vi "CreatePrivateEvents.vi"(8 "error in (no error)":errorcluster, 11 "LockinDAQ":refnum<class "LockinDAQ.lvclass">) -> (0 "error out":errorcluster, 3 "LockinDAQ out":refnum<class "LockinDAQ.lvclass">)   [LabVIEW 2016, in "LockinDAQ.lvclass"]
doc: "---------------------------------------------------------------\nJKI State Machine Objects™\nhttp://jki.net/state-machine-objects/\nCopyright (C) 2005-2015, JKI <info@jki.net>\nALL RIGHTS RESERVEDJKI State Machine Objects (SMO) 1.0.0.4\nJKI - JKI\nCopyright (c) 2015, JKI"
uses:
  LockinDAQ.lvclass
  Typedefs/PrivateEvents--LockinDAQ.setAOconfig.ctl
  Typedefs/AO.config-array.ctl
  Typedefs/AO.config-cluster.ctl
  Typedefs/446xAO-enum.ctl
  Typedefs/PrivateEvents--LockinDAQ.setAIconfig.ctl
  Typedefs/AI.config-array.ctl
  Typedefs/AI.config-cluster.ctl
  Typedefs/AI.coupling-enum.ctl
  Typedefs/446xAI-enum.ctl
  Typedefs/PrivateEvents--LockinDAQ.setAO.ctl
  Typedefs/AO-cluster.ctl
  Typedefs/AO_Amp-array.ctl
  Typedefs/AO_DC-array.ctl
  Typedefs/AO_f-array.ctl
  Typedefs/AO_phi-array.ctl
  Typedefs/Function-array.ctl
  Typedefs/Function-enum.ctl
  Typedefs/PrivateEvents--LockinDAQ.setREF.ctl
  Typedefs/REF-cluster.ctl
  Typedefs/REF_f-array.ctl
  Typedefs/REF_phi-array.ctl
  Typedefs/PrivateEvents--LockinDAQ.setSampling.ctl
  Typedefs/Sampling.ctl
  Typedefs/PrivateEvents--LockinDAQ.setState.ctl
  Typedefs/Set State-enum.ctl
  LockinDAQ.lvclass/LockinDAQ.ctl
  <vilib>/JKI/JKI SMO/SMO/SMO.lvclass
panel:
  # "For instructions on how to use the JKI State Machine Objects, examples and video tutorials, visit:\nhttp://jki.net/state-machine-objects/\n\nJKI State Machine Objects™\nhttp://jki.net/state-machine-objects/\nCopyright (C) 2005-2015, JKI <info@jki.net>\nALL RIGHTS RESERVED"
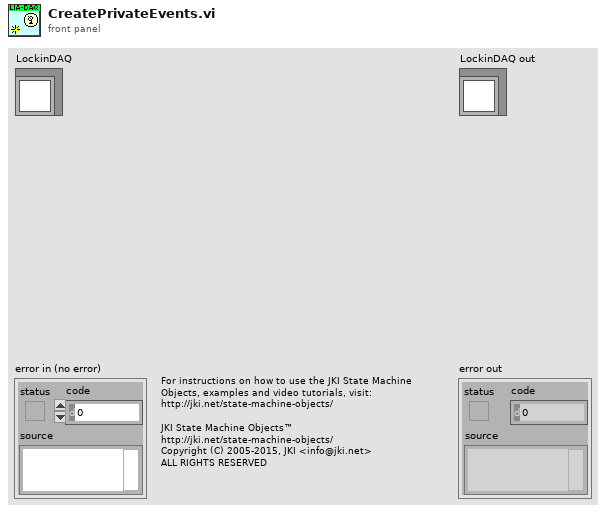
[diagram p1: front panel]
types:
  T1 = typedef "LockinDAQ.lvclass/PrivateEvents--LockinDAQ.setState.ctl" = cluster{"setState":T2}
  T2 = typedef "LockinDAQ.lvclass/Set State-enum.ctl" = enum16{"start", "stop", "reset"}
  T3 = typedef "LockinDAQ.lvclass/PrivateEvents--LockinDAQ.setSampling.ctl" = cluster{"sampling":T4, "sample mode":i32}
  T4 = typedef "Sampling.ctl" = cluster{"Fs":dbl, "#s":i32}
  T5 = typedef "LockinDAQ.lvclass/PrivateEvents--LockinDAQ.setREF.ctl" = cluster{"Channels: Lockin":T6}
  T6 = typedef "REF-cluster.ctl" = cluster{"REF f (Hz)":T7, "REF phi (°)":T8}
  T7 = typedef "REF_f-array.ctl" = dbl[]
  T8 = typedef "REF_phi-array.ctl" = dbl[]
  T9 = typedef "LockinDAQ.lvclass/PrivateEvents--LockinDAQ.setAO.ctl" = cluster{"Channels: AO":T10}
  T10 = typedef "AO-cluster.ctl" = cluster{"AO amp (V)":T11, "AO DC (V)":T12, "AO f (Hz)":T13, "AO phi (°)":T14, "function":T15, "I+":bool[]}
  T11 = typedef "AO_Amp-array.ctl" = dbl[]
  T12 = typedef "AO_DC-array.ctl" = dbl[]
  T13 = typedef "AO_f-array.ctl" = dbl[]
  T14 = typedef "AO_phi-array.ctl" = dbl[]
  T15 = typedef "Function-array.ctl" = T16[]
  T16 = typedef "Function-enum.ctl" = enum16{"Sine", "Triangle", "Square", "Sawtooth"}
  T17 = typedef "LockinDAQ.lvclass/PrivateEvents--LockinDAQ.setAIconfig.ctl" = cluster{"AI Configuration":T18}
  T18 = typedef "AI.config-array.ctl" = T19[]
  T19 = typedef "AI.config-cluster.ctl" = cluster{"AI.Coupling":T20, "AI.channels":tag, "AI.Range":T21}
  T20 = typedef "AI.coupling-enum.ctl" = enum16{"AC", "DC", "GND"}
  T21 = typedef "446xAI-enum.ctl" = enum16{"±0.316 V", "±1.00 V", "±3.16 V", "±10.0 V", "±31.6 V", "±42.4 V"}
  T22 = typedef "LockinDAQ.lvclass/PrivateEvents--LockinDAQ.setAOconfig.ctl" = cluster{"AO Configuration":T23}
  T23 = typedef "AO.config-array.ctl" = T24[]
  T24 = typedef "AO.config-cluster.ctl" = cluster{"AO.Range":T25, "AO.channels":tag}
  T25 = typedef "446xAO-enum.ctl" = enum16{"±0.1 V", "±1.0 V", "±10.0 V"}
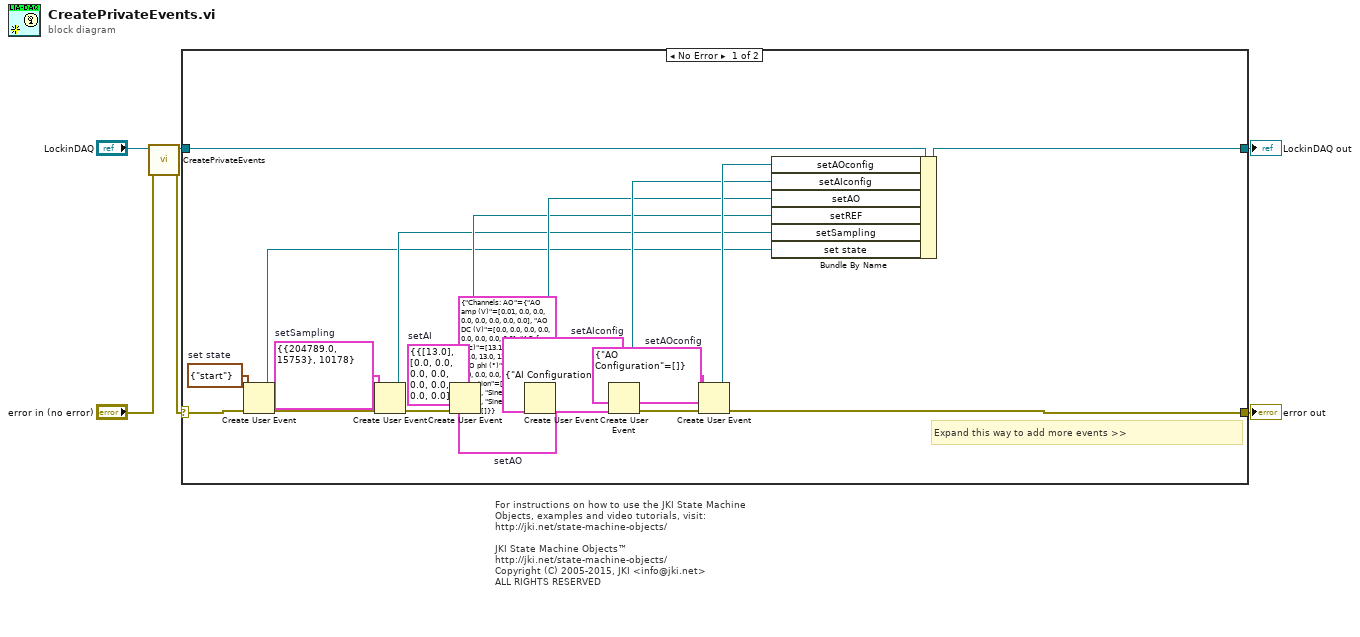
[diagram p0: block diagram]
diagram:
  # "For instructions on how to use the JKI State Machine Objects, examples and video tutorials, visit:\nhttp://jki.net/state-machine-objects/\n\nJKI State Machine Objects™\nhttp://jki.net/state-machine-objects/\nCopyright (C) 2005-2015, JKI <info@jki.net>\nALL RIGHTS RESERVED"
  n1 = call-parent "CreatePrivateEvents.vi"("error in (no error)"="error in (no error)", "SMO"="LockinDAQ") -> ("error out"=w1:errorcluster, "SMO out"=w3:refnum<class "LockinDAQ.lvclass">)  [unwired: 8 in]
  n2 = case shown="No Error" w1 {
    selector: w1 -> [w26 w29]
    tunnel: [w24 w29] -> w5
    tunnel: [w25 w28] -> w6
    tunnel: w3 -> [w27 w28]
    frame No Error {
      w8 = T1 {"setState"=enum."start"}  # set state
      w11 = T3 {"sampling"={"Fs"=204789.0, "#s"=15753}, "sample mode"=10178}  # setSampling
      w14 = T5 {"Channels: Lockin"={"REF f (Hz)"=[13.0], "REF phi (°)"=[0.0, 0.0, 0.0, 0.0, 0.0, 0.0, 0.0, 0.0]}}  # setAI
      w17 = T9 {"Channels: AO"={"AO amp (V)"=[0.01, 0.0, 0.0, 0.0, 0.0, 0.0, 0.0, 0.0], "AO DC (V)"=[0.0, 0.0, 0.0, 0.0, 0.0, 0.0, 0.0, 0.0], "AO f (Hz)"=[13.1, 13.0, 13.0, 13.0, 13.0, 13.0, 13.0, 13.0], "AO phi (°)"=[0.0, 0.0, 0.0, 0.0, 0.0, 0.0, 0.0, 0.0], "function"=[enum."Sine", enum."Sine", enum."Sine", enum."Sine", enum."Sine", enum."Sine", enum."Sine", enum."Sine"], "I+"=[]}}  # setAO
      w20 = T17 {"AI Configuration"=[]}  # setAIconfig
      w23 = T22 {"AO Configuration"=[]}  # setAOconfig
      # "Expand this way to add more events >>"
      n3 = Create User Event(user event datatype=w8, error in=w26) -> (user event=w7:refnum<user-event>, error out=w9:errorcluster)
      n4 = Create User Event(user event datatype=w11, error in=w9) -> (user event=w10:refnum<user-event>, error out=w12:errorcluster)
      n5 = Create User Event(user event datatype=w14, error in=w12) -> (user event=w13:refnum<user-event>, error out=w15:errorcluster)
      n6 = Create User Event(user event datatype=w17, error in=w15) -> (user event=w16:refnum<user-event>, error out=w18:errorcluster)
      n7 = Create User Event(user event datatype=w20, error in=w18) -> (user event=w19:refnum<user-event>, error out=w21:errorcluster)
      n8 = Create User Event(user event datatype=w23, error in=w21) -> (user event=w22:refnum<user-event>, error out=w24:errorcluster)
      n9 = Bundle By Name(cluster=w27, "setAOconfig"=w22, "setAIconfig"=w19, "setAO"=w16, "setREF"=w13, "setSampling"=w10, "set state"=w7) -> (w25:refnum<class "LockinDAQ.lvclass">)
    }
    frame Error {
    }
  }
  "error out" <- w5
  "LockinDAQ out" <- w6
